vi "ma_Basic Averaged DC-RMS no state.vi"(5 "reset":bool, 6 "state info":T1 {"buffer" format="%0.2f"; "timestamp" format="%<%.4X>T"; "dt history" format="%0.2f"; "t0 history" format="%<%I:%M:%S%4u %p>T"; "exp TC (samples)" format="%0.2f"; "RMS history" format="%0.2f"; "DC history" format="%0.2f"}, 8 "error in":errorcluster, 9 "window":T2(ring), 10 "averaging type":enum16{"Linear", "Exponential"}(ring), 11 "signal in":waveform(dbl)) -> (0 "error out":errorcluster, 1 "measurement info cluster":T3 {"uncertainty" format="%0.2p"}, 2 "RMS value":dbl format="%0.2p", 3 "DC value":dbl format="%0.2p", 4 "state info":T1 {"buffer" format="%0.2f"; "timestamp" format="%<%.4X>T"; "dt history" format="%0.2f"; "t0 history" format="%<%I:%M:%S%4u %p>T"; "exp TC (samples)" format="%0.2f"; "RMS history" format="%0.2f"; "DC history" format="%0.2f"})   [LabVIEW 2022 SP3, in "NI_MAPro.lvlib"]
doc: "This VI takes a signal in, applies a window to the signal, and averages the DC and RMS values calculated from the windowed signal with the previous DC and RMS values according to the averaging type input."
uses:
  NI_MAPro.lvlib
panel:
  # "Single Point\nAveraged DC-RMS"
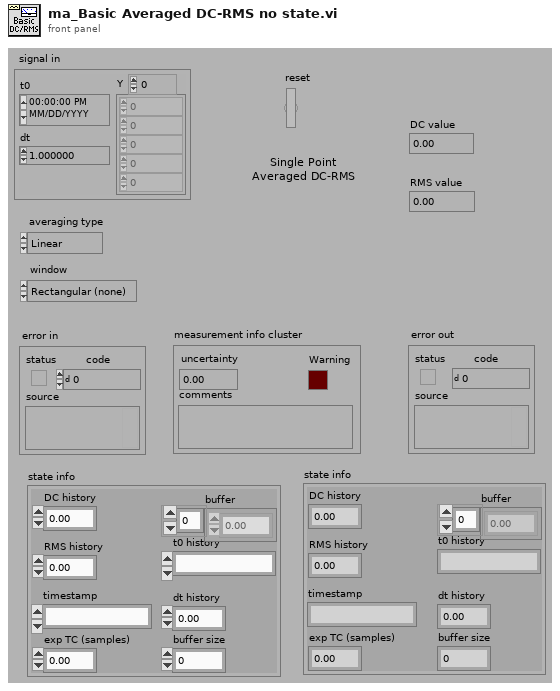
[diagram p1: front panel]
types:
  T1 = cluster{"DC history":dbl, "RMS history":dbl, "exp TC (samples)":dbl, "buffer size":i32, "t0 history":timestamp, "dt history":dbl, "timestamp":timestamp, "buffer":dbl[]}
  T2 = enum16{"Rectangular (none)", "Hanning", "Low side lobe"}
  T3 = cluster{"uncertainty":dbl, "Warning":bool, "comments":string}
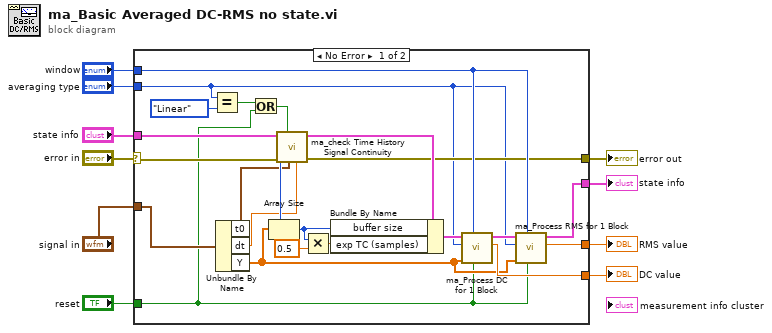
[diagram p0: block diagram]
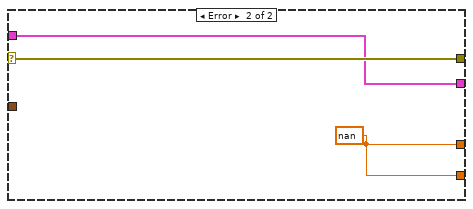
[diagram p2: hidden frame]
diagram:
  n1 = case shown="No Error" "error in" {
    selector: "error in" -> [w19 w35]
    tunnel: [w18 w35] -> w10
    tunnel: [w27 w34] -> w8
    tunnel: [w22 w34] -> w2
    tunnel: "averaging type" -> [w14 _]
    tunnel: "signal in" -> [w31 _]
    tunnel: "window" -> [w32 _]
    tunnel: "reset" -> [w12 _]
    tunnel: "state info" -> [w26 w33]
    tunnel: [w21 w33] -> w1
    frame No Error {
      n2 = Equal?(x=w14, y=enum16{"Linear", "Exponential"}."Linear" ("averaging type")) -> (x = y?=w13:bool)
      n3 = Unbundle By Name(w31) -> ("t0"=w16:timestamp, "dt"=w17:dbl, "Y"=w23:dbl[])
      n4 = Or(x=w13, y=w12) -> (x .or. y?=w11:bool)
      n5 = Array Size(array=w23) -> (size(s)=w24:i32)
      n6 = call "ma_check Time History Signal Continuity.vi"("dt"=w17, "t0"=w16, "Ignore input start time"=w11, "error in (no error)"=w19, "# samples"=w24, "state info"=w26) -> ("error out"=w18:errorcluster, "state info"=w25:T1)  [unwired: 1 in, 3 out]
      n7 = Multiply(x=w24, y=0.5) -> (x*y=w29:dbl)
      n8 = Bundle By Name(cluster=w25, "buffer size"=w24, "exp TC (samples)"=w29) -> (w28:T1)
      n9 = call "ma_Process DC for 1 Block.vi"("reset"=w12, "window for DC"=w32, "time signal data (samples)"=w23, "averaging type"=w14, "state info"=w28) -> ("DC value data"=w27:dbl, "state info"=w20:T1)  [unwired: 5 in]
      n10 = call "ma_Process RMS for 1 Block.vi"("reset"=w12, "window for RMS"=w32, "time signal data (samples)"=w23, "averaging type"=w14, "state info"=w20) -> ("RMS value data"=w22:dbl, "state info"=w21:T1)  [unwired: 5 in]
    }
    frame Error {
      w34 = nan ("DC value data")
    }
  }
  "error out" <- w10
  "DC value" <- w8
  "RMS value" <- w2
  "state info" <- w1
